vi "Write Scanner driver.vi"(8 "error in (no error)":errorcluster, 10 "Channel Scanner Driver.lvclass":refnum<class "Channel Scanner Driver.lvclass">, 11 "Channel Scanner in":refnum<class "Channel Scanner.lvclass">) -> (0 "error out":errorcluster, 3 "Channel Scanner out":refnum<class "Channel Scanner.lvclass">)   [LabVIEW 2016, in "Channel Scanner.lvclass"]
uses:
  Channel Scanner.lvclass
  C:/github/LabActor/Instrument Actor/Instrument Actor.lvclass
  NHMFL_Core/Libraries/Instruments/Instrument Driver/Channel Scanner Driver/Channel Scanner Driver.lvclass
  C:/github/NHMFL_Core/Libraries/Instruments/Instrument Driver/Instrument Driver.lvclass
  Instrument Actor/Instrument Actor.lvclass/Instrument Actor.ctl
  Instrument Actor/Write Instrument driver.vi
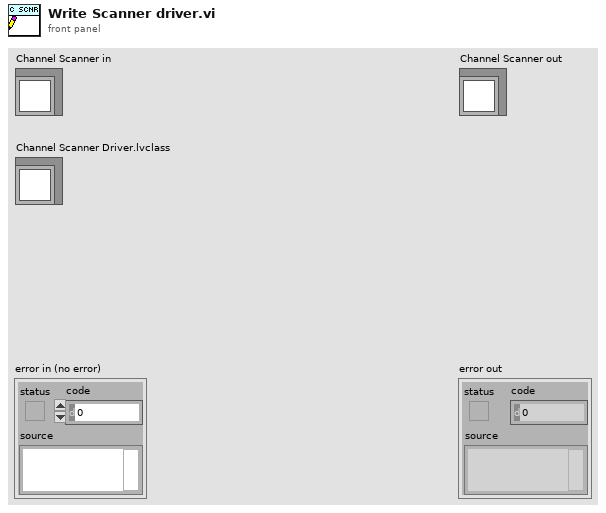
[diagram p1: front panel]
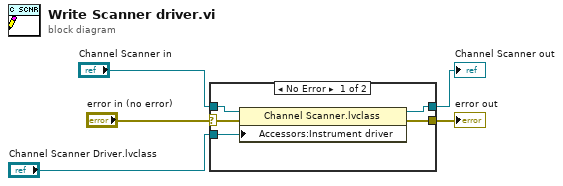
[diagram p0: block diagram]
diagram:
  n1 = case shown="No Error" "error in (no error)" {
    selector: "error in (no error)" -> [w7 w11]
    tunnel: [w6 w11] -> w4
    tunnel: [w9 w12] -> w2
    tunnel: "Channel Scanner in" -> [w10 w12]
    tunnel: "Channel Scanner Driver.lvclass" -> [w8 _]
    frame No Error {
      n2 = property class="Channel Scanner.lvclass"(reference=w10, error in=w7, "Accessors:Instrument driver"=w8) -> (reference out=w9:refnum<class "Channel Scanner.lvclass">, error out=w6:errorcluster)
    }
    frame Error {
    }
  }
  "error out" <- w4
  "Channel Scanner out" <- w2
